vi "create default alias.vi"(8 "error in":errorcluster, 11 "configuration in":refnum<class "NISE_CEF_serializable configuration.lvclass">) -> (0 "error out":errorcluster, 2 "default alias":string, 3 "configuration out":refnum<class "NISE_CEF_serializable configuration.lvclass">)   [LabVIEW 2013, in "NISE_CEF_serializable configuration.lvclass"]
uses:
  NISE_CEF_serializable configuration.lvclass
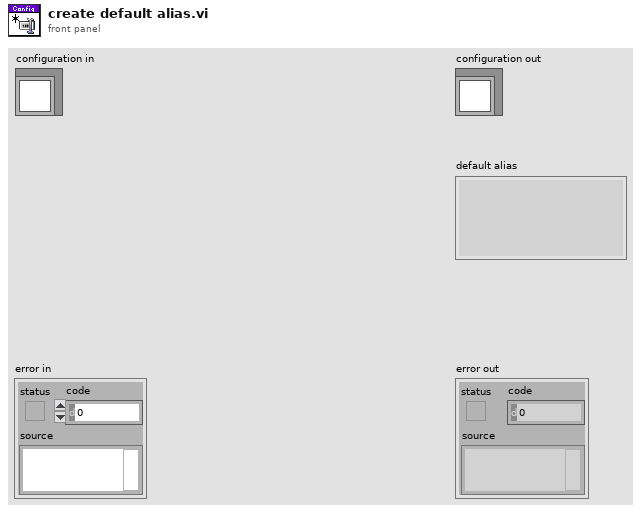
[diagram p1: front panel]
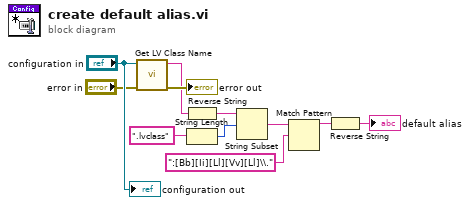
[diagram p0: block diagram]
diagram:
  n1 = call <vilib>:"Get LV Class Name.vi"("error in (no error)"="error in", "object"="configuration in") -> ("error out"=→"error out":errorcluster, "class name"=w8:string)  [unwired: 8 in]
  n2 = Reverse String(1:w8) -> (0:w7:string)
  n3 = String Length(string=".lvclass") -> (length=w5:i32)
  n4 = String Subset(string=w7, offset (0)=w5) -> (substring=w4:string)  [unwired: 1 in]
  n5 = Match Pattern(string=w4, regular expression=":[Bb][Ii][Ll][Vv][Ll]\\.") -> (before substring=w2:string)  [unwired: 1 in, 3 out]
  n6 = Reverse String(1:w2) -> (0:→"default alias":string)
  "configuration out" <- "configuration in"
